vi "PM9_TCP_READ-DEV-STATUS.vi"(0 "VISA":refnum<visa-resource-name>="TCPIP0::169.254.70.190::502::SOCKET", 5 "connection ID":refnum<k5>, 11 "error in (no error)":errorcluster, 14 "Close tcp(t)":bool) -> (3 "Dev OK(t)":bool, 4 "visa out":refnum<visa-resource-name>, 6 "connection ID out":refnum<k5>, 15 "error out":errorcluster)   [LabVIEW 2018]
panel:
  # "Use a valid connection id to run in loop"
  # "1\t1\t16\t1016\t1\tDEV\t\t\t(none)\t\tDevice Status\tMonitor the controller's status for hardware failure.\tOK (138), Fail (32)\tno default\tEnumeration\tR\t30\t400,031\tN/A\t0 to 40\t0x65\t101\t1\t16\t1"
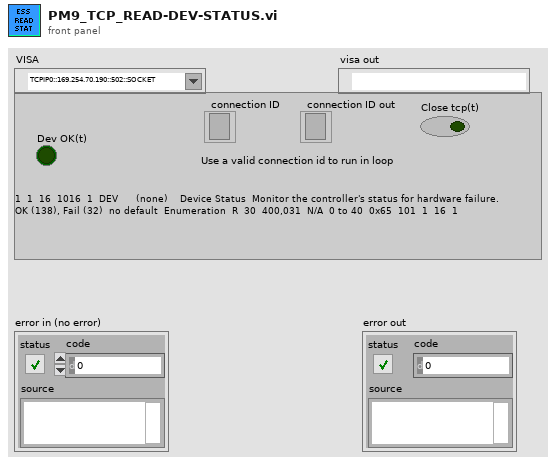
[diagram p1: front panel]
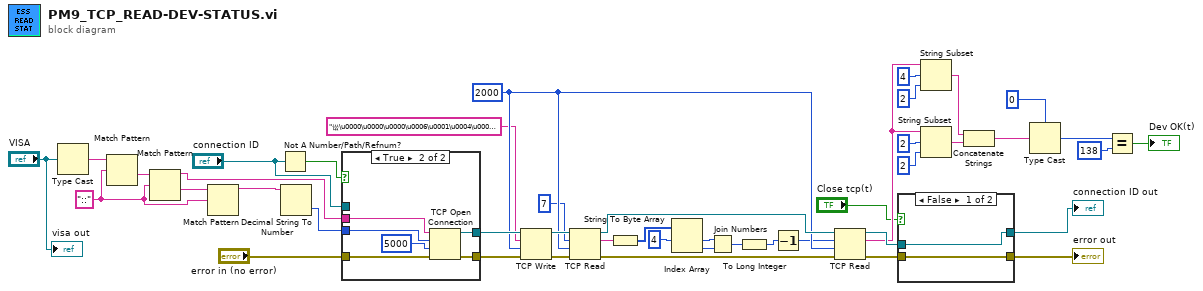
[diagram p0: block diagram]
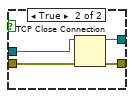
[diagram p3: hidden frame]
diagram:
  w13 = "::" ("search string/char (-)")
  w37 = 2000 ("timeout ms (25000)")
  n1 = Type Cast(x="VISA") -> (*(type *) &x=w16:string)  [unwired: 1 in]
  n2 = Match Pattern(string=w16, regular expression=w13) -> (after substring=w15:string)  [unwired: 1 in, 3 out]
  n3 = Match Pattern(string=w15, regular expression=w13) -> (before substring=w11:string, after substring=w14:string)  [unwired: 1 in, 2 out]
  n4 = Match Pattern(string=w14, regular expression=w13) -> (before substring=w12:string)  [unwired: 1 in, 3 out]
  n5 = Not A Number/Path/Refnum?(number/path/refnum="connection ID") -> (NaN/Path/Refnum?=w5:bool)
  n6 = Decimal String To Number(string=w12) -> (number=w10:i32)  [unwired: 2 in, 1 out]
  n7 = case shown="True" w5 {
    tunnel: [w47 w53] -> w45
    tunnel: [w46 w52] -> w44
    tunnel: w11 -> [_ w50]
    tunnel: w10 -> [_ w49]
    tunnel: "error in (no error)" -> [w46 w48]
    tunnel: "connection ID" -> [w47 _]
    frame False {
    }
    frame True {
      n8 = TCP Open Connection(address=w50, remote port or service name=w49, timeout ms (60000)=5000, error in (no error)=w48) -> (connection ID=w53:refnum<k5>, error out=w52:errorcluster)  [unwired: 1 in]
    }
  }
  n9 = TCP Write(connection ID=w45, data in="讼\u0000\u0000\u0000\u0006\u0001\u0004\u0000\u001e\u0000\u0002" ("address"), error in (no error)=w44, 9:w37) -> (connection ID out=w41:refnum<k5>, error out=w39:errorcluster)  [unwired: 1 out]
  n10 = TCP Read(connection ID=w41, bytes to read=7, error in (no error)=w39, 9:w37) -> (connection ID out=w40:refnum<k5>, data out=w29:string, error out=w38:errorcluster)  [unwired: 1 in]
  n11 = String To Byte Array(string=w29) -> (unsigned byte array=w30:u8[])
  n12 = Index Array(array=w30, index #1=4 ("index")) -> (element #1=w31:u8, element #2=w32:u8)  [unwired: 1 in]
  n13 = Join Numbers(hi=w31, lo=w32) -> ((hi.lo)=w34:u16)
  n14 = To Long Integer(number=w34) -> (32bit integer=w33:i32)
  n15 = Decrement(x=w33) -> (x-1=w28:i32)
  n16 = TCP Read(connection ID=w40, bytes to read=w28, error in (no error)=w38, 9:w37) -> (connection ID out=w43:refnum<k5>, data out=w22:string, error out=w42:errorcluster)  [unwired: 1 in]
  n17 = case shown="False" "Close tcp(t)" {
    tunnel: w43 -> [w55 w59]
    tunnel: w42 -> [w54 w58]
    tunnel: [w54 w57] -> w1
    tunnel: [w55 w56] -> w8
    frame False {
    }
    frame True {
      n18 = TCP Close Connection(connection ID=w59, error in (no error)=w58) -> (connection ID out=w56:refnum<k5>, error out=w57:errorcluster)  [unwired: 1 in]
    }
  }
  "error out" <- w1
  "connection ID out" <- w8
  n19 = String Subset(string=w22, offset (0)=u16 4 ("bytes to read"), length (rest)=u16 2 ("bytes to read")) -> (substring=w21:string)
  n20 = String Subset(string=w22, offset (0)=u16 2 ("bytes to read"), length (rest)=u16 2 ("bytes to read")) -> (substring=w20:string)
  n21 = Concatenate Strings(w21, w20) -> (w19:string)
  n22 = Type Cast(type=0 ("bytes to read"), x=w19) -> (*(type *) &x=w4:i32)
  n23 = Equal?(x=w4, y=138) -> (x = y?=→"Dev OK(t)":bool)
  "visa out" <- "VISA"
